vi "Agilent VNA Read Trigger Mode.vi"(6 "Channel":i8=1 min=1 max=99 step=1, 7 "Agilent VNA":T1, 8 "error in (no error)":errorcluster, 11 "VISA Resource Name":refnum<visa-resource-name>) -> (0 "error out":errorcluster, 2 "Trigger Mode":T2, 3 "dup VISA Resource Name":refnum<visa-resource-name>)   [LabVIEW 2011]
doc: "This VI for the HP8753B Network Analyzers reads the stimulus values. Except when performing log sweeps and freq list sweeps, this VI uses the start and stop values and the number of points to calcuate the stimulus values."
uses:
  TypeDefs/Agilent VNA Trigger Mode.ctl
  TypeDefs/Agilent VNA Instrument Info.ctl
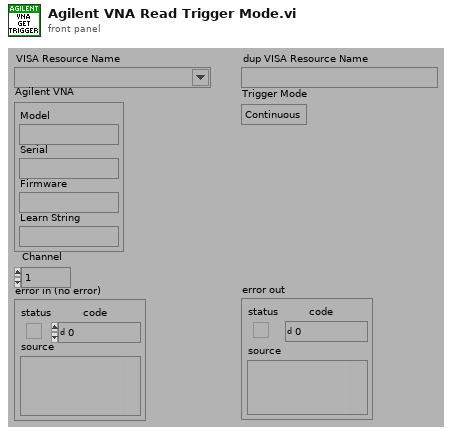
[diagram p1: front panel]
types:
  T1 = typedef "Agilent VNA Instrument Info.ctl" = cluster{"Model":string, "Serial":string, "Firmware":string, "Learn String":string}
  T2 = typedef "Agilent VNA Trigger Mode.ctl" = enum16{"Continuous", "Hold", "Single"}
  T3 = typedef "Agilent VNA Model.ctl" = enum16{"Not Supported", "8510X", "8719X", "8720X", "8722X", "8753X", "ENA", "PNA", "Field Fox"}
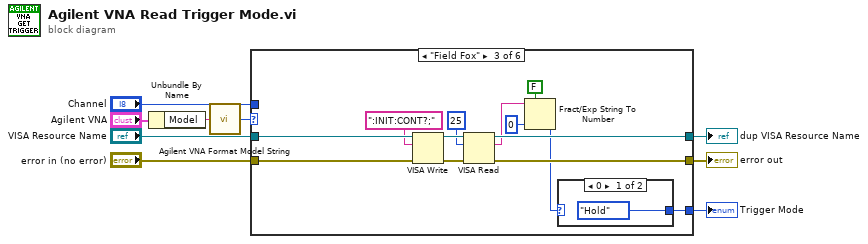
[diagram p0: block diagram]
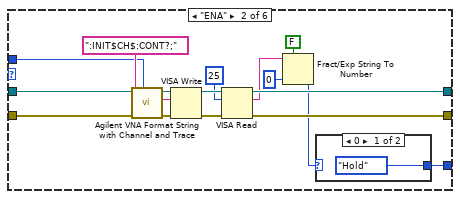
[diagram p3: hidden frame]
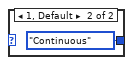
[diagram p4: hidden frame]
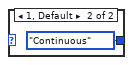
[diagram p5: hidden frame]
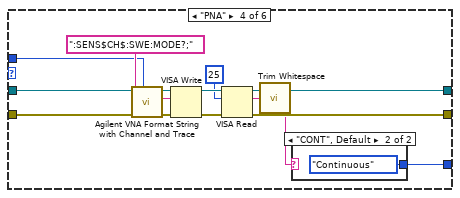
[diagram p6: hidden frame]
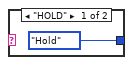
[diagram p7: hidden frame]
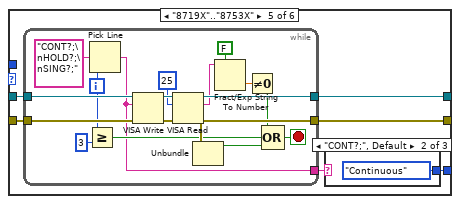
[diagram p8: hidden frame]
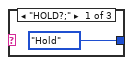
[diagram p9: hidden frame]
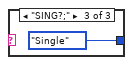
[diagram p10: hidden frame]
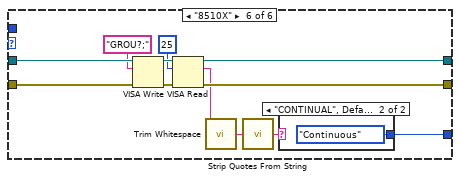
[diagram p11: hidden frame]
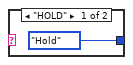
[diagram p12: hidden frame]
diagram:
  n1 = Unbundle By Name("Agilent VNA") -> ("Model"=w1:string)
  n2 = call "Agilent VNA Format Model String.vi"("Model"=w1) -> ("Model"=w4:T3)
  n3 = case shown="\"Field Fox\"" w4 {
    tunnel: "error in (no error)" -> [w11 w26 w41 w56 w64 w97]
    tunnel: [w11 w24 w39 w54 w63 w96] -> w8
    tunnel: "VISA Resource Name" -> [w10 w21 w36 w51 w62 w95]
    tunnel: [w10 w23 w38 w53 w61 w94] -> w6
    tunnel: [_ w15 w30 w49 w60 w93] -> w5
    tunnel: "Channel" -> [_ w12 _ w44 _ _]
    frame "Not Supported" {
    }
    frame "ENA" {
      n4 = call "Agilent VNA Format String with Channel and Trace.vi"("Channel"=w12, "String"=":INIT$CH$:CONT?;") -> ("String Out"=w13:string)  [unwired: 1 in, 6 out]
      n5 = VISA Write(VISA resource name=w21, write buffer=w13, error in (no error)=w26) -> (VISA resource name out=w22:refnum<visa-resource-name>, error out=w25:errorcluster)  [unwired: 1 out]
      n6 = VISA Read(VISA resource name=w22, byte count=u32 25, error in (no error)=w25) -> (VISA resource name out=w23:refnum<visa-resource-name>, read buffer=w18:string, error out=w24:errorcluster)  [unwired: 1 out]
      n7 = Fract/Exp String To Number(use system decimal point (T)=FALSE, string=w18, default (0 dbl)=0 ("default (0 DBL)")) -> (number=w16:i32)  [unwired: 2 out]
      n8 = case shown="0" w16 {
        tunnel: [Agilent_VNA_Trigger_Mode."Hold" Agilent_VNA_Trigger_Mode."Continuous"] -> w15
        frame 0 {
        }
        frame 1, Default {
        }
      }
    }
    frame "Field Fox" {
      n9 = VISA Write(VISA resource name=w36, write buffer=":INIT:CONT?;", error in (no error)=w41) -> (VISA resource name out=w37:refnum<visa-resource-name>, error out=w40:errorcluster)  [unwired: 1 out]
      n10 = VISA Read(VISA resource name=w37, byte count=u32 25, error in (no error)=w40) -> (VISA resource name out=w38:refnum<visa-resource-name>, read buffer=w33:string, error out=w39:errorcluster)  [unwired: 1 out]
      n11 = Fract/Exp String To Number(use system decimal point (T)=FALSE, string=w33, default (0 dbl)=0 ("default (0 DBL)")) -> (number=w31:i32)  [unwired: 2 out]
      n12 = case shown="0" w31 {
        tunnel: [Agilent_VNA_Trigger_Mode."Hold" Agilent_VNA_Trigger_Mode."Continuous"] -> w30
        frame 0 {
        }
        frame 1, Default {
        }
      }
    }
    frame "PNA" {
      n13 = call "Agilent VNA Format String with Channel and Trace.vi"("Channel"=w44, "String"=":SENS$CH$:SWE:MODE?;") -> ("String Out"=w47:string)  [unwired: 1 in, 6 out]
      n14 = VISA Write(VISA resource name=w51, write buffer=w47, error in (no error)=w56) -> (VISA resource name out=w52:refnum<visa-resource-name>, error out=w55:errorcluster)  [unwired: 1 out]
      n15 = VISA Read(VISA resource name=w52, byte count=u32 25, error in (no error)=w55) -> (VISA resource name out=w53:refnum<visa-resource-name>, read buffer=w46:string, error out=w54:errorcluster)  [unwired: 1 out]
      n16 = call <vilib>:"Trim Whitespace.vi"("string"=w46) -> ("trimmed string"=w45:string)  [unwired: 1 in]
      n17 = case shown="\"CONT\", Default" w45 {
        tunnel: [Agilent_VNA_Trigger_Mode."Hold" Agilent_VNA_Trigger_Mode."Continuous"] -> w49
        frame "HOLD" {
        }
        frame "CONT", Default {
        }
      }
    }
    frame "8719X".."8753X" {
      n18 = while {
        tunnel: w64 -> [w85]
        tunnel: [w81] -> w63
        tunnel: w62 -> [w84]
        tunnel: [w80] -> w61
        tunnel: [w68] -> w59
        i -> [w74]
        stop <- w69 stop-if-true
        n19 = Greater Or Equal?(x=w74, y=3) -> (x >= y?=w70:bool)
        n20 = Pick Line(multi-line string="CONT?;\nHOLD?;\nSING?;", line index=w74) -> (output string=w68:string)  [unwired: 1 out]
        n21 = VISA Write(VISA resource name=w84, write buffer=w68, error in (no error)=w85) -> (VISA resource name out=w83:refnum<visa-resource-name>, error out=w82:errorcluster)  [unwired: 1 out]
        n22 = VISA Read(VISA resource name=w83, byte count=u32 25, error in (no error)=w82) -> (VISA resource name out=w80:refnum<visa-resource-name>, read buffer=w77:string, error out=w81:errorcluster)  [unwired: 1 out]
        n23 = Unbundle(w81) -> ("status"=w71:bool)  [unwired: 2 out]
        n24 = Fract/Exp String To Number(use system decimal point (T)=FALSE, string=w77) -> (number=w75:dbl)  [unwired: 3 out]
        n25 = Not Equal To 0?(x=w75) -> (x != 0?=w72:bool)
        n26 = Compound Arithmetic op=OR(w72, w70, w71) -> (w69:bool)
      }
      n27 = case shown="\"CONT?;\", Default" w59 {
        tunnel: [Agilent_VNA_Trigger_Mode."Hold" Agilent_VNA_Trigger_Mode."Continuous" Agilent_VNA_Trigger_Mode."Single"] -> w60
        frame "HOLD?;" {
        }
        frame "CONT?;", Default {
        }
        frame "SING?;" {
        }
      }
    }
    frame "8510X" {
      n28 = VISA Write(VISA resource name=w95, write buffer="GROU?;", error in (no error)=w97) -> (VISA resource name out=w92:refnum<visa-resource-name>, error out=w91:errorcluster)  [unwired: 1 out]
      n29 = VISA Read(VISA resource name=w92, byte count=u32 25, error in (no error)=w91) -> (VISA resource name out=w94:refnum<visa-resource-name>, read buffer=w86:string, error out=w96:errorcluster)  [unwired: 1 out]
      n30 = call <vilib>:"Trim Whitespace.vi"("string"=w86) -> ("trimmed string"=w87:string)  [unwired: 1 in]
      n31 = call "Strip Quotes From String.vi"("String In"=w87) -> ("Trimmed String"=w88:string)
      n32 = case shown="\"CONTINUAL\", Default" w88 {
        tunnel: [Agilent_VNA_Trigger_Mode."Hold" Agilent_VNA_Trigger_Mode."Continuous"] -> w93
        frame "HOLD" {
        }
        frame "CONTINUAL", Default {
        }
      }
    }
  }
  "dup VISA Resource Name" <- w6
  "error out" <- w8
  "Trigger Mode" <- w5
